vi "OAT Locate Waveform Segment for Unfiltered Data.vi"(9 "revolutions to display":cluster{"start (rev)":dbl, "revolutions":dbl}={"start (rev)"=0.0, "revolutions"=1.0} {"revolutions" format="%.2f"; "start (rev)" format="%.2f"}, 10 "pulse/revolution (1)":i32=1, 11 "pulse positions [s]":dbl[](array[numeric]) format="%.2f") -> (0 "last point":dbl format="%.2f", 1 "durations":dbl[](array[numeric]), 2 "duration":dbl format="%.2f", 3 "start points":dbl[](array[numeric]) format="%.2f")   [LabVIEW 2017]
uses:
  <vilib>/Analysis/2dsp.llb/Decimate (single shot, DBL).vi
  <vilib>/Analysis/NI_AALPro.lvlib
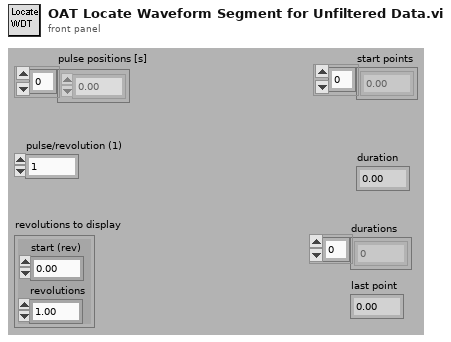
[diagram p1: front panel]
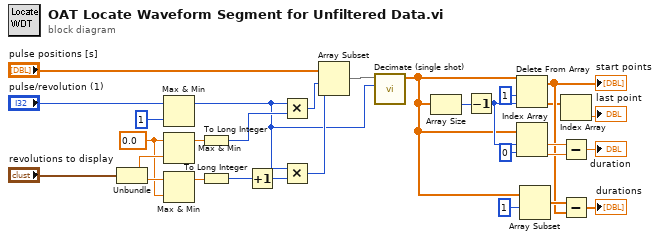
[diagram p0: block diagram]
diagram:
  w22 = 0.0 ("y")
  n1 = Unbundle("revolutions to display") -> ("start (rev)"=w29:dbl, "revolutions"=w24:dbl)
  n2 = Max & Min(x="pulse/revolution (1)", y=1) -> (max(x,y)=w19:i32)  [unwired: 1 out]
  n3 = Max & Min(x=w22, y=w29) -> (max(x,y)=w28:dbl)  [unwired: 1 out]
  n4 = Max & Min(x=w24, y=w22) -> (max(x,y)=w23:dbl)  [unwired: 1 out]
  n5 = To Long Integer(number=w28) -> (32bit integer=w20:i32)
  n6 = To Long Integer(number=w23) -> (32bit integer=w17:i32)
  n7 = Increment(x=w17) -> (x+1=w16:i32)
  n8 = Multiply(x=w19, y=w20) -> (x*y=w14:i32)
  n9 = Multiply(x=w19, y=w16) -> (x*y=w21:i32)
  n10 = Array Subset(array="pulse positions [s]", index=w14, length=w21) -> (w30:dbl[])
  n11 = call-poly <vilib>:"Decimate (single shot).vi"("decimating factor"=w19, "X"=w30) -> ("Decimated Array"=w7:dbl[])  [unwired: 8 in, 1 out]
  n12 = Array Size(array=w7) -> (size(s)=w18:i32)
  n13 = Decrement(x=w18) -> (x-1=w12:i32)
  n14 = Delete From Array(array=w7, length=1 ("index"), index=w12) -> (deleted portion=w2:dbl[], array with subset deleted=w4:dbl[])
  "start points" <- w4
  n15 = Index Array(array=w7, index #1=w12, index #2=0 ("index")) -> (element #1=w10:dbl, element #2=w9:dbl)
  n16 = Array Subset(array=w7, index=1) -> (w5:dbl[])  [unwired: 1 in]
  n17 = Index Array(array=w2) -> (element=→"last point":dbl)  [unwired: 1 in]
  n18 = Subtract(x=w10, y=w9) -> (x-y=→"duration":dbl)
  n19 = Subtract(x=w5, y=w4) -> (x-y=→"durations":dbl[])
